vi "Init.vi"(8 "error in (no error)":errorcluster, 9 "Config File Path":path=path "", 10 "Name":string, 11 "Execution API In":refnum<class "Execution API.lvclass">) -> (0 "error out":errorcluster, 3 "Execution API Out":refnum<class "Execution API.lvclass">)   [LabVIEW 2020, in "Execution API.lvclass"]
doc: "Initializes the process and creates necessary references. Anything initialized here is released in the Clear.vi method."
uses:
  Execution API.lvclass
  Test Runner/Test Runner.lvclass
  C:/Git/astemes-lunit/source/Application Framework/Process Classes/Process/Process.lvclass
  Report Generator/Report Generator.lvclass
  Result Collector/Result Collector.lvclass
  Helper Classes/Buffered Test Finder/Indexing Test Finder.lvclass
  C:/Git/astemes-lunit/source/Framework/Helper Classes/Test Finder/Test Finder.lvclass
  Application Framework/Process Classes/Error Handler/Error Handler.lvclass
  Helper Classes/Buffered Test Finder/Indexing Test Finder.lvclass/Indexing Test Finder.ctl
  Report Generator/Report Generator.lvclass/Report Generator.ctl
  Application Framework/Process Classes/Process/Process.lvclass/Process.ctl
  Execution API.lvclass/Execution API.ctl
  Application Framework/Process Classes/Process/Protected/Messaging/Enqueue Message.vi
  Application Framework/Process Classes/Process/Process.lvclass
  C:/Git/astemes-lunit/source/Framework/Helper Classes/Open Test Case Interface/Open Test Case.lvclass
  C:/Git/astemes-lunit/source/Framework/Helper Classes/Buffered Test Finder/Indexing Test Finder.lvclass
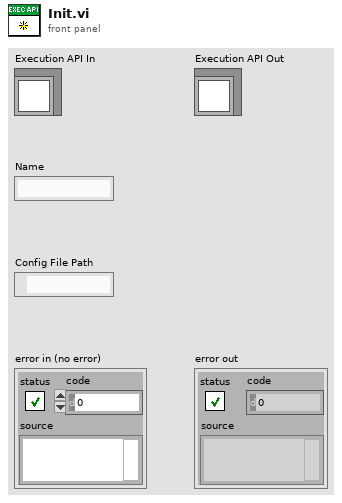
[diagram p1: front panel]
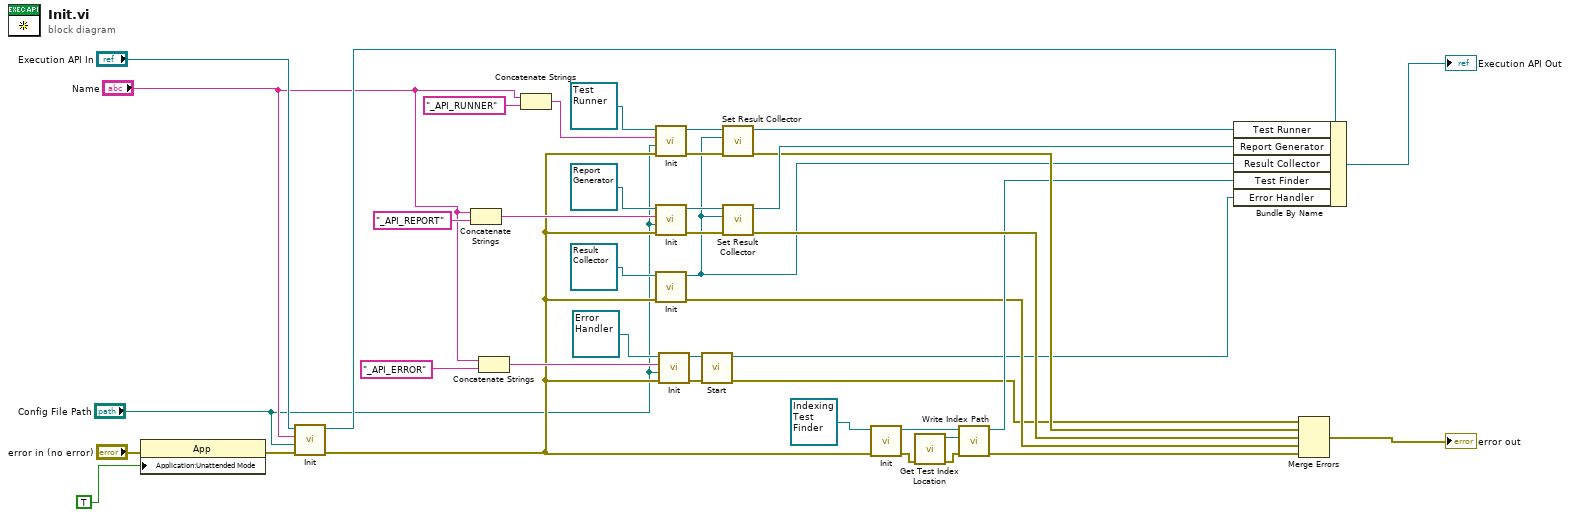
[diagram p0: block diagram]
diagram:
  n1 = property class="App"(error in="error in (no error)", "Application:Unattended Mode"=TRUE) -> (error out=w11:errorcluster)  [unwired: 1 in, 1 out]
  n2 = call-parent "Init.vi"("error in (no error)"=w11, "Config File Path"="Config File Path", "Name"="Name", "Process In"="Execution API In") -> ("error out"=w4:errorcluster, "Process Out"=w36:refnum<class "Execution API.lvclass">)  [unwired: 6 in]
  n3 = Concatenate Strings("Name", "_API_REPORT") -> (w32:string)
  n4 = Concatenate Strings("Name", "_API_ERROR") -> (w5:string)
  n5 = Concatenate Strings("Name", "_API_RUNNER") -> (w34:string)
  n6 = call-dynamic "Init.vi"("error in (no error)"=w4, "Config File Path"="Config File Path", "Name"=w34, "Test Runner In"=refnum<class "Test Runner.lvclass"> refnum ("Test Runner.lvclass")) -> ("error out"=w23:errorcluster, "Test Runner Out"=w26:refnum<class "Test Runner.lvclass">)  [unwired: 6 in]
  n7 = call-dynamic "Init.vi"("error in (no error)"=w4, "Config File Path"="Config File Path", "Name"=w32, "Report Generator In"=refnum<class "Report Generator.lvclass"> refnum ("Test Report Generator.lvclass")) -> ("error out"=w29:errorcluster, "Report Generator Out"=w31:refnum<class "Report Generator.lvclass">)  [unwired: 6 in]
  n8 = call-dynamic "Init.vi"("error in (no error)"=w4, "Report Generator In"=refnum<class "Result Collector.lvclass"> refnum ("Result Collector.lvclass")) -> ("error out"=w14:errorcluster, "Report Generator Out"=w22:refnum<class "Result Collector.lvclass">)  [unwired: 8 in]
  n9 = call-dynamic "Init.vi"("error in (no error)"=w4, "Configuration File Path"="Config File Path", "Process Name"=w5, "Error Handler In"=refnum<class "Error Handler.lvclass"> refnum ("Error Handler in")) -> ("error out"=w8:errorcluster, "Error Handler Out"=w9:refnum<class "Error Handler.lvclass">)  [unwired: 6 in]
  n10 = call "Start.vi"("error in (no error)"=w8, "Process In"=w9) -> ("error out"=w2:errorcluster, "Process Out"=w1:refnum<class "Error Handler.lvclass">)  [unwired: 8 in]
  n11 = call "Set Result Collector.vi"("error in (no error)"=w23, "Result Collector"=w22, "Test Runner In"=w26) -> ("error out"=w24:errorcluster, "Test Runner Out"=w25:refnum<class "Test Runner.lvclass">)  [unwired: 7 in]
  n12 = call "Set Result Collector.vi"("error in (no error)"=w29, "Result Collector.lvclass"=w22, "Report Generator in"=w31) -> ("error out"=w28:errorcluster, "Report Generator out"=w30:refnum<class "Report Generator.lvclass">)  [unwired: 7 in]
  n13 = call-dynamic "Init.vi"("error in (no error)"=w4, "Test Finder in"=refnum<class "Indexing Test Finder.lvclass"> refnum ("Test Finder")) -> ("error out"=w17:errorcluster, "Test Finder out"=w20:refnum<class "Indexing Test Finder.lvclass">)  [unwired: 8 in]
  n14 = call "Get Test Index Location.vi"("error in (no error)"=w17) -> ("error out"=w16:errorcluster, "Test Index Location"=w15:path)  [unwired: 9 in]
  n15 = call "Write Index Path.vi"("error in (no error)"=w16, "Index Folder Path"=w15, "Indexing Test Finder in"=w20) -> ("error out"=w18:errorcluster, "Indexing Test Finder out"=w19:refnum<class "Indexing Test Finder.lvclass">)  [unwired: 7 in]
  n16 = Bundle By Name(cluster=w36, "Test Runner"=w25, "Report Generator"=w30, "Result Collector"=w22, "Test Finder"=w19, "Error Handler"=w1) -> (→"Execution API Out":refnum<class "Execution API.lvclass">)
  n17 = Merge Errors(w2, w24, w28, w14, w18) -> (→"error out":errorcluster)
